vi "Unbenannt 1.vi"() -> ()   [LabVIEW 2013]
panel:
  out "Daten":i32
  in  "Stopp":bool
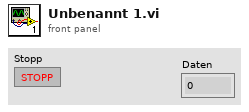
[diagram p1: front panel]
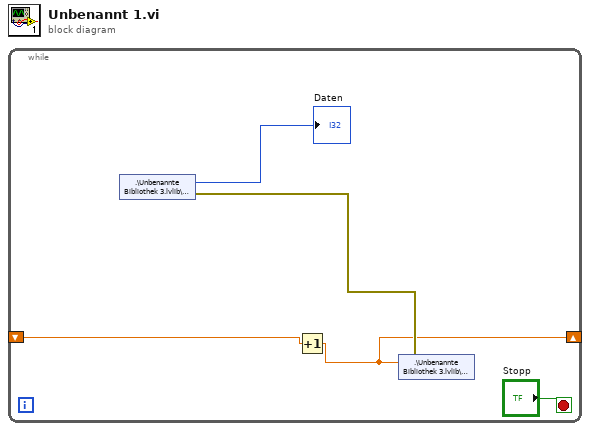
[diagram p0: block diagram]
diagram:
  n1 = while {
    shift-right: [w2] -> _
    shift-left: _ -> [w1]
    stop <- "Stopp" stop-if-true
    n2 = shared-variable ".\\Unbenannte Bibliothek 3.lvlib\\Daten"() -> (→"Daten":u32, error out=w4:errorcluster)  [unwired: 1 in]
    n3 = Increment(x=w1) -> (x+1=w2:dbl)
    n4 = shared-variable ".\\Unbenannte Bibliothek 3.lvlib\\Daten"(w2, error in=w4) -> ()  [unwired: 1 out]
  }
